vi "UpdatePSF.vi"(4 "Gaussian Profile?":bool, 5 "Edge Roll-off (dB)":dbl=10.0, 6 "Powers of 2 higher":i32=1, 7 "Window":T2=enum."Hamming", 8 "Zero-Pad the FFT?":bool, 9 "Index of Refraction":dbl=1.0 format="%_3g", 10 "Spacing (GHz)":dbl=0.1 format="%_6g", 11 "Interferometer":dbl[](array[numeric])) -> (0 "Phase Angle (rad)":dbl[](array[numeric]), 1 "X-resolution (mm)":dbl, 2 "PSF DataOut":T1, 3 "FFT":cluster{dbl[], dbl[]}(graph))   [LabVIEW 2015]
doc: "This VI analyzes an interferogram and produces the PSF and statistics about the strongest reflection in the data set.\n\nINPUTS\n1) Interferometer data\n2) Sample Pt Spacing (GHz)\n3) Index of Refraction - default is 1.0\n4) FFT control parameters\n 4.1) Apply a Gaussian Profile to the Time Record?\n 4.2) Edge Roll-off to apply to the Gaussian Profile (dB)\n 4.3) Window to apply to the Time Record (done after the Gaussian profile)\n 4.4) Zero-pad the time record?\n 4.5) What power of 2 higher to zero pad the time record length\n\n\nOUTPUTS\nPSF = 20*Log(Ampl) vs. X-position\nPhase = phase angle (wrapped) at each frequency bin / x-position, radians\nFW@3dB = Full-Width at 3-dB down\nFW@20dB = Full-Width at 20-dB down\nYpeak = Maximum amplitude in the PSF, in dB.\nXpeak = Location of the maximum amplitude, in mm.\nPTSR = Peak-To-Sidelobe Ratio\nPNFR = Peak-to-Noise-Floor Ratio\nWLRange (GHz) = calculated sweep range in GHz"
uses:
  Window_Functions.ctl
  <vilib>/Analysis/4window.llb/Gaussian Window (DBL).vi
  <vilib>/Analysis/4window.llb/Hanning Window (DBL).vi
  <vilib>/Analysis/4window.llb/Blackman-Harris Window (DBL).vi
  <vilib>/Analysis/4window.llb/Hamming Window (DBL).vi
  <vilib>/Analysis/4window.llb/Blackman Window (DBL).vi
  <vilib>/Analysis/4window.llb/Kaiser-Bessel Window (DBL).vi
  <vilib>/Analysis/2dsp.llb/Real FFT.vi
  <vilib>/Analysis/baseanly.llb/Mean (DBL).vi
  <vilib>/Analysis/4window.llb/AllCosWindow (DBL).vi
  <vilib>/measure/matone.llb/Extract Single Tone Information 1 Chan.vi
  <vilib>/Utility/file.llb/Write To Spreadsheet File (DBL).vi
  <vilib>/Analysis/NI_AALPro.lvlib
  <vilib>/measure/NI_MAPro.lvlib
  <vilib>/Analysis/NI_AAL_SigProc.lvlib
  <vilib>/Analysis/NI_AALBase.lvlib
panel:
  in  "Pts to skip":i32=4
  out "PNFR (dB)":dbl
  out "Noise Floor (dB)":dbl format="%0.2f"
  out "Side-Lobe Location (mm)":dbl
  out "Side-Lobe Amp (dB)":dbl
  out "Xpeak":dbl
  out "Ypeak":dbl
  out "FW@20dB":dbl
  out "FW@3dB":dbl
  in  "PSFData":path=path "I:/BTDemo/PSFData.txt"
  out "PTSR (dB)":dbl
  out "Period (pts)":dbl
  out "Amplitude":dbl
  out "Freq (1/pts)":dbl
  in  "Save Data":bool
  out "Interferometer Signal":dbl[](graph)
  # "UpdatePSF"
  # "PSF Peak Finding"
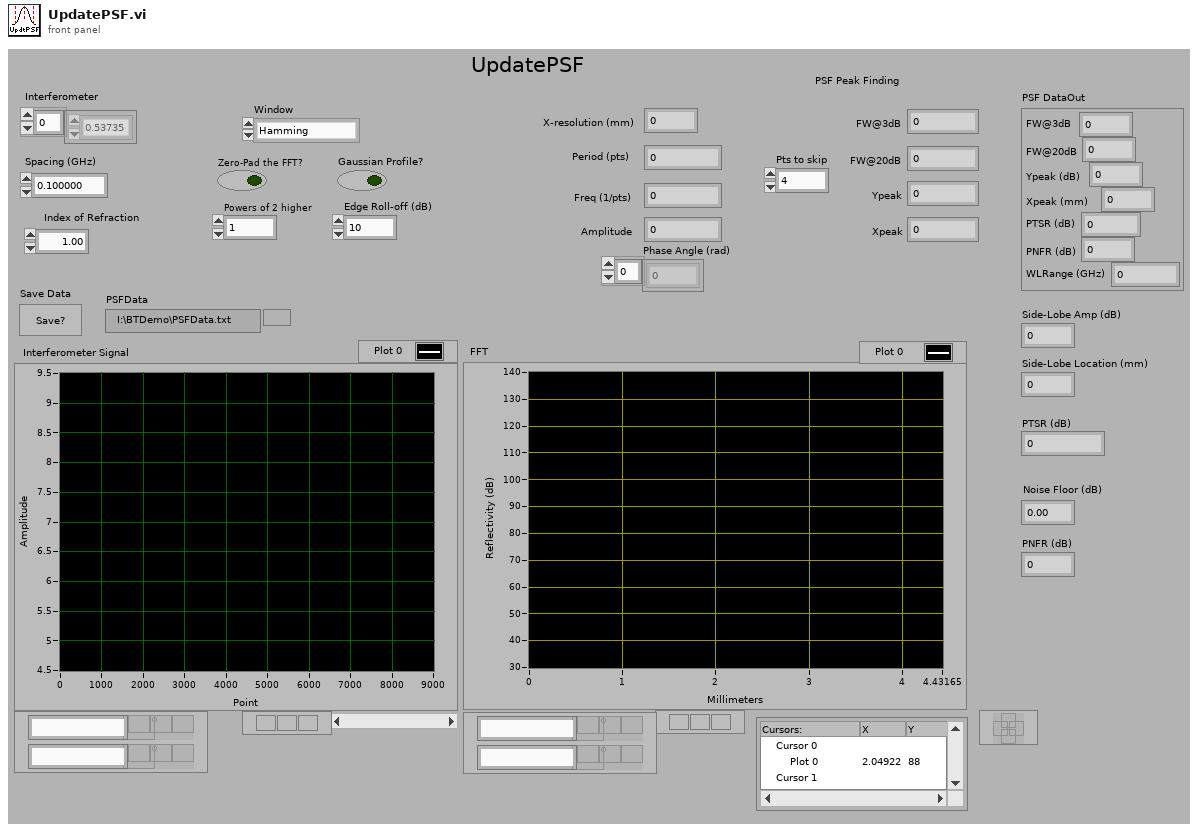
[diagram p1: front panel]
types:
  T1 = cluster{"FW@3dB":dbl, "FW@20dB":dbl, "Ypeak (dB)":dbl, "Xpeak (mm)":dbl, "PTSR (dB)":dbl, "PNFR (dB) ":dbl, "WLRange (GHz)":dbl}
  T2 = typedef "Window_Functions.ctl" = enum16{"Rectangular", "Hann", "Hamming", "Blackman", "Blackman-Harris", "Kaiser 7", "Kaiser 14"}
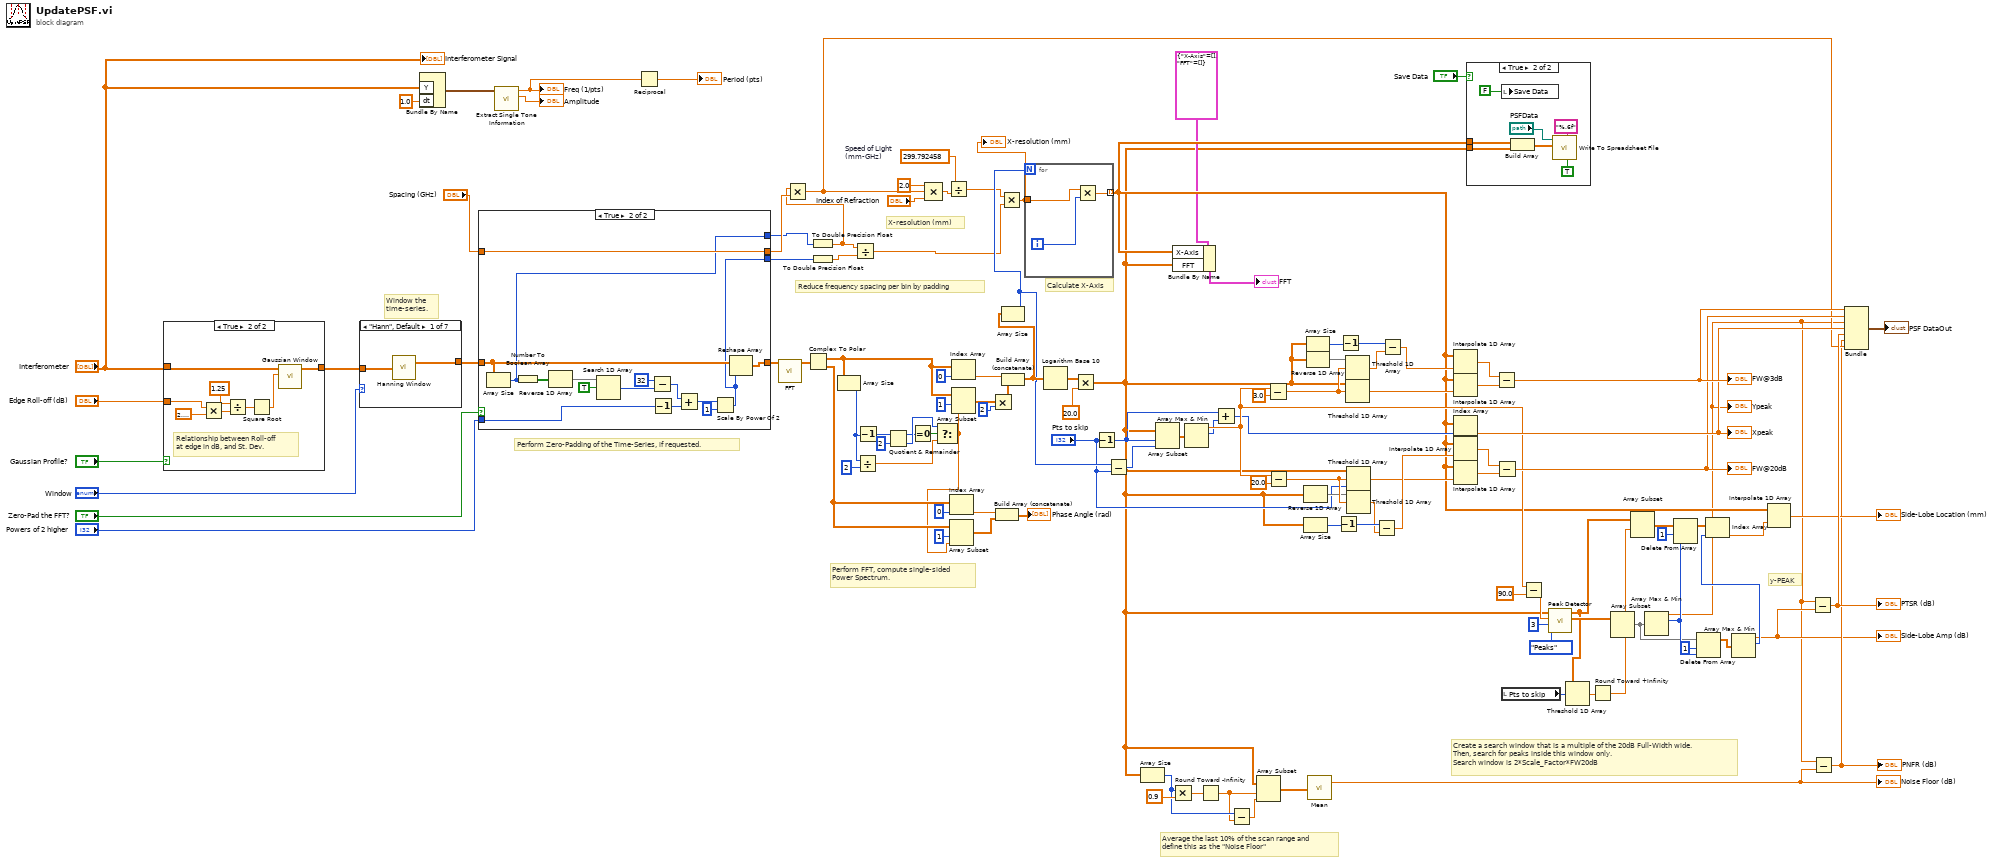
[diagram p0: block diagram]
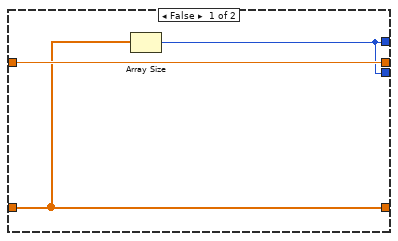
[diagram p3: hidden frame]
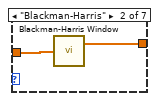
[diagram p5: hidden frame]
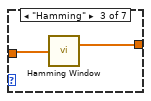
[diagram p6: hidden frame]
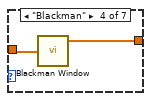
[diagram p7: hidden frame]
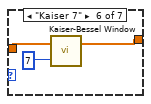
[diagram p9: hidden frame]
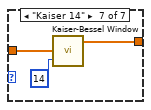
[diagram p10: hidden frame]
diagram:
  w70 = 299.792458  # Speed of Light  (mm-GHz)
  # "Reduce frequency spacing per bin by padding"
  # "Average the last 10% of the scan range and \ndefine this as the \"Noise Floor\""
  # "Create a search window that is a multiple of the 20dB Full-Width wide.\nThen, search for peaks inside this window only.\nSearch window is 2*Scale_Factor*FW20dB"
  # "X-resolution (mm)"
  # "y-PEAK"
  # "Perform FFT, compute single-sided\nPower Spectrum."
  # "Window the \ntime-series."
  # "Perform Zero-Padding of the Time-Series, if requested."
  # "Calculate X-Axis"
  n1 = case shown="True" "Gaussian Profile?" {
    tunnel: [w122 w125] -> w39
    tunnel: "Interferometer" -> [w122 w124]
    tunnel: "Edge Roll-off (dB)" -> [_ w123]
    frame False {
    }
    frame True {
      # "Relationship between Roll-off \nat edge in dB, and St. Dev."
      n2 = Multiply(x=w123, y=2.302585092994046) -> (x*y=w128:dbl)
      n3 = Divide(x=1.25, y=w128) -> (x/y=w130:dbl)
      n4 = Square Root(x=w130) -> (sqrt(x)=w126:dbl)
      n5 = call-poly <vilib>:"Gaussian Window.vi"("standard deviation"=w126, "X"=w124) -> ("Windowed X"=w125:dbl[])  [unwired: 8 in, 1 out]
    }
  }
  n6 = case shown="\"Hann\", Default" "Window" {
    tunnel: [w132 w134 w135 w137 w139 w141 w145] -> w101
    tunnel: w39 -> [w131 w133 w136 w138 w139 w142 w144]
    frame "Hann", Default {
      n7 = call-poly <vilib>:"Hanning Window.vi"("X"=w131) -> ("Windowed X"=w132:dbl[])  [unwired: 1 out]
    }
    frame "Blackman-Harris" {
      n8 = call-poly <vilib>:"Blackman-Harris Window.vi"("X"=w133) -> ("Windowed X"=w134:dbl[])  [unwired: 1 out]
    }
    frame "Hamming" {
      n9 = call-poly <vilib>:"Hamming Window.vi"("X"=w136) -> ("Windowed X"=w135:dbl[])  [unwired: 1 out]
    }
    frame "Blackman" {
      n10 = call-poly <vilib>:"Blackman Window.vi"("X"=w138) -> ("Windowed X"=w137:dbl[])  [unwired: 1 out]
    }
    frame "Rectangular" {
    }
    frame "Kaiser 7" {
      n11 = call-poly <vilib>:"Kaiser-Bessel Window.vi"("beta"=7, "X"=w142) -> ("Windowed X"=w141:dbl[])  [unwired: 1 out]
    }
    frame "Kaiser 14" {
      n12 = call-poly <vilib>:"Kaiser-Bessel Window.vi"("beta"=14, "X"=w144) -> ("Windowed X"=w145:dbl[])  [unwired: 1 out]
    }
  }
  n13 = Bundle By Name("Y"="Interferometer", "dt"=1.0) -> (w114:waveform(dbl))  [unwired: 1 in]
  n14 = case shown="True" "Zero-Pad the FFT?" {
    tunnel: [w147 w163] -> w100
    tunnel: "Powers of 2 higher" -> [_ w157]
    tunnel: w101 -> [w147 w153]
    tunnel: "Spacing (GHz)" -> [w148 w151]
    tunnel: [w148 w151] -> w68
    tunnel: [w146 w150] -> w21
    tunnel: [w146 w149] -> w15
    frame False {
      n15 = Array Size(array=w147) -> (size(s)=w146:i32)
    }
    frame True {
      n16 = Array Size(array=w153) -> (size(s)=w150:i32)
      n17 = Number To Boolean Array(number=w150) -> (Boolean array=w161:bool[])
      n18 = Reverse 1D Array(array=w161) -> (reversed array=w160:bool[])
      n19 = Search 1D Array(1D array=w160, element=TRUE) -> (index of element=w159:i32)  [unwired: 1 in]
      n20 = Subtract(x=32, y=w159) -> (x-y=w156:i32)
      n21 = Decrement(x=w157) -> (x-1=w152:i32)
      n22 = Add(x=w156, y=w152) -> (x+y=w155:i32)
      n23 = Scale By Power Of 2(n=w155, x=1) -> (x*2^n=w149:i32)
      n24 = Reshape Array(w153, w149) -> (w163:dbl[])
    }
  }
  n25 = call-poly <vilib>:"Extract Single Tone Information.vi"("time signal in"=w114) -> ("detected amplitude"=→"Amplitude":dbl, "detected frequency"=w111:dbl)  [unwired: 5 in, 4 out]
  "Freq (1/pts)" <- w111
  n26 = Reciprocal(x=w111) -> (1/x=→"Period (pts)":dbl)
  n27 = call-poly <vilib>:"FFT.vi"("X"=w100) -> ("FFT {X}"=w36:cdb[])  [unwired: 9 in, 1 out]
  n28 = Complex To Polar(r * e^(i*theta)=w36) -> (r=w35:dbl[], theta=w29:dbl[])
  n29 = To Double Precision Float(number=w21) -> (double precision float=w19:dbl)
  n30 = Multiply(x=w19, y=w68) -> (x*y=w50:dbl)
  n31 = To Double Precision Float(number=w15) -> (double precision float=w20:dbl)
  n32 = Array Size(array=w35) -> (size(s)=w69:i32)
  n33 = Divide(x=w19, y=w20) -> (x/y=w16:dbl)
  n34 = Divide(x=w69, y=2) -> (x/y=w99:dbl)
  n35 = Decrement(x=w69) -> (x-1=w93:i32)
  n36 = Quotient & Remainder(x=w93, y=2) -> (x-y*floor(x/y)=w95:i32, floor(x/y)=w97:i32)
  n37 = Equal To 0?(x=w95) -> (x = 0?=w96:bool)
  n38 = Compound Arithmetic op=MULTIPLY(2.0, w50, "Index of Refraction") -> (w71:dbl)
  n39 = Select(t=w97, s=w96, f=w99) -> (s? t:f=w28:dbl)
  n40 = Divide(x=w70, y=w71) -> (x/y=w18:dbl)
  n41 = Index Array(array=w29, index=0) -> (element=w32:dbl)
  n42 = Array Subset(array=w29, index=1, length=w28) -> (w31:dbl[])
  n43 = Index Array(array=w35, index=0) -> (element=w119:dbl)
  n44 = Array Subset(array=w35, index=1, length=w28) -> (w118:dbl[])
  n45 = Multiply(x=w118, y=2) -> (x*y=w116:dbl[])
  n46 = Build Array (concatenate)(w32, w31) -> (→"Phase Angle (rad)":dbl[])
  n47 = Multiply(x=w18, y=w16) -> (x*y=w17:dbl)
  "X-resolution (mm)" <- w17
  n48 = Build Array (concatenate)(w119, w116) -> (w67:dbl[])
  n49 = Array Size(array=w67) -> (size(s)=w22:i32)
  n50 = for {
    N: w22 -> [_]
    tunnel: [w166] -> w14 mode=indexing
    tunnel: w17 -> [w164]
    i -> [w165]
    n51 = Multiply(x=w164, y=w165) -> (x*y=w166:dbl)
  }
  n52 = Logarithm Base 10(1:w67) -> (0:w110:dbl[])
  n53 = Multiply(x=w110, y=20.0) -> (x*y=w10:dbl[])
  n54 = Decrement(x="Pts to skip") -> (x-1=w24:i32)
  n55 = Subtract(x=w22, y="Pts to skip") -> (x-y=w26:i32)
  n56 = Array Size(array=w10) -> (size(s)=w53:i32)
  n57 = Array Subset(array=w10, index=w24, length=w26) -> (w27:dbl[])
  n58 = Multiply(x=w53, y=0.9) -> (x*y=w52:dbl)
  n59 = Bundle By Name(cluster=cluster{"X-Axis":dbl[], "FFT":dbl[]} {"X-Axis"=[], "FFT"=[]}, "X-Axis"=w14, "FFT"=w10) -> (→"FFT":cluster{"X-Axis":dbl[], "FFT":dbl[]})
  n60 = Array Max & Min(array=w27) -> (max value=w56:dbl, max index (indices)=w25:i32)  [unwired: 2 out]
  n61 = Round Toward -Infinity(1:w52) -> (0:w51:dbl)
  n62 = Add(x=w24, y=w25) -> (x+y=w23:i32)
  n63 = Subtract(x=w53, y=w51) -> (x-y=w54:dbl)
  n64 = Array Subset(array=w10, index=w51, length=w54) -> (w57:dbl[])
  n65 = Subtract(x=w56, y=3.0) -> (x-y=w85:dbl)
  n66 = Subtract(x=w56, y=20.0) -> (x-y=w80:dbl)
  n67 = Reverse 1D Array(array=w10) -> (reversed array=w79:dbl[])
  n68 = Array Size(array=w10) -> (size(s)=w77:i32)
  n69 = Array Size(array=w10) -> (size(s)=w82:i32)
  n70 = Reverse 1D Array(array=w10) -> (reversed array=w86:dbl[])
  n71 = call-poly <vilib>:"Mean.vi"("X"=w57) -> ("mean"=w55:dbl)  [unwired: 1 out]
  "Noise Floor (dB)" <- w55
  n72 = Decrement(x=w77) -> (x-1=w78:i32)
  n73 = Decrement(x=w82) -> (x-1=w81:i32)
  n74 = Threshold 1D Array(2:w85, 3:w86) -> (0:w84:dbl)  [unwired: 1 in]
  n75 = Threshold 1D Array(2:w85, 3:w10) -> (0:w62:dbl)  [unwired: 1 in]
  n76 = Threshold 1D Array(1:"Pts to skip", 2:w80, 3:w10) -> (0:w60:dbl)
  n77 = Threshold 1D Array(2:w80, 3:w79) -> (0:w76:dbl)  [unwired: 1 in]
  n78 = Subtract(x=w78, y=w76) -> (x-y=w61:dbl)
  n79 = Subtract(x=w81, y=w84) -> (x-y=w63:dbl)
  n80 = Interpolate 1D Array(1:w63, 2:w14) -> (0:w83:dbl)
  n81 = Interpolate 1D Array(1:w62, 2:w14) -> (0:w90:dbl)
  n82 = Index Array(array=w14, index=w23) -> (element=w74:dbl)
  "Xpeak" <- w74
  n83 = Interpolate 1D Array(1:w61, 2:w14) -> (0:w88:dbl)
  n84 = Interpolate 1D Array(1:w60, 2:w14) -> (0:w89:dbl)
  n85 = case shown="True" "Save Data" {
    tunnel: w14 -> [_ w169]
    tunnel: w10 -> [_ w168]
    frame False {
    }
    frame True {
      n86 = local write "Save Data"(FALSE) -> ()
      n87 = Build Array(w169, w168) -> (w171:dbl[][])
      n88 = call-poly <vilib>:"Write To Spreadsheet File.vi"("transpose? (no:F)"=TRUE, "format (%.3f)"="%.6f", "2D data"=w171, "file path (dialog if empty)"="PSFData") -> ()  [unwired: 4 in, 1 out]
    }
  }
  n89 = Subtract(x=w83, y=w90) -> (x-y=w75:dbl)
  "FW@3dB" <- w75
  n90 = Subtract(x=w88, y=w89) -> (x-y=w73:dbl)
  "FW@20dB" <- w73
  n91 = local read "Pts to skip"() -> (w1:i32)
  n92 = Subtract(x=w56, y=90.0) -> (x-y=w64:dbl)
  n93 = call <vilib>:"Peak Detector.vi"("peaks/valleys"=enum32{"Peaks", "Valleys"}."Peaks", "width"=3, "threshold"=w64, "X"=w10) -> ("Amplitudes"=w7:dbl[], "Locations"=w3:dbl[])  [unwired: 3 in, 3 out]
  n94 = Threshold 1D Array(2:w1, 3:w3) -> (0:w4:dbl)  [unwired: 1 in]
  n95 = Round Toward +Infinity(x=w4) -> (ceil(x): smallest int >= x=w2:dbl)
  n96 = Array Subset(array=w7, index=w2) -> (w6:dbl[])  [unwired: 1 in]
  n97 = Array Subset(array=w3, index=w2) -> (w5:dbl[])  [unwired: 1 in]
  n98 = Array Max & Min(array=w6) -> (max value=w9:dbl, max index (indices)=w42:i32)  [unwired: 2 out]
  "Ypeak" <- w9
  n99 = Delete From Array(array=w5, length=1, index=w42) -> (array with subset deleted=w45:dbl[])  [unwired: 1 out]
  n100 = Delete From Array(array=w6, length=1, index=w42) -> (array with subset deleted=w43:dbl[])  [unwired: 1 out]
  n101 = Array Max & Min(array=w43) -> (max value=w41:dbl, max index (indices)=w44:i32)  [unwired: 2 out]
  "Side-Lobe Amp (dB)" <- w41
  n102 = Index Array(array=w45, index=w44) -> (element=w8:dbl)
  n103 = Interpolate 1D Array(1:w8, 2:w14) -> (0:→"Side-Lobe Location (mm)":dbl)
  n104 = Subtract(x=w9, y=w41) -> (x-y=w106:dbl)
  "PTSR (dB)" <- w106
  n105 = Subtract(x=w9, y=w55) -> (x-y=w49:dbl)
  "PNFR (dB)" <- w49
  n106 = Bundle(w75, w73, w9, w74, w106, w49, w50) -> (→"PSF DataOut":cluster{dbl, dbl, dbl, dbl, dbl, dbl, dbl})  [unwired: 1 in]
  "Interferometer Signal" <- "Interferometer"
